vi "Read PWM Ratio.vi"(8 "error in (no error)":errorcluster, 11 "Set Ratio Msg in":refnum<class "Set Ratio Msg.lvclass">) -> (0 "error out":errorcluster, 2 "PWM Ratio":dbl format="%.3g", 3 "Set Ratio Msg out":refnum<class "Set Ratio Msg.lvclass">)   [LabVIEW 2017, in "BNT_DAQmx.lvlib" / "Set Ratio Msg.lvclass"]
uses:
  Set Ratio Msg.lvclass
  Set Ratio Msg.lvclass/Set Ratio Msg.ctl
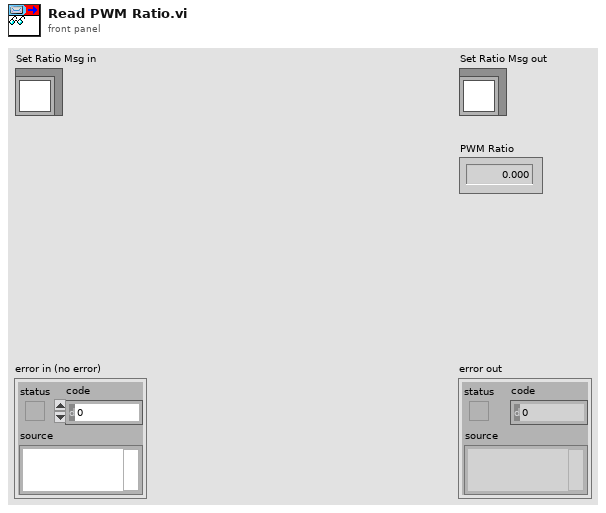
[diagram p1: front panel]
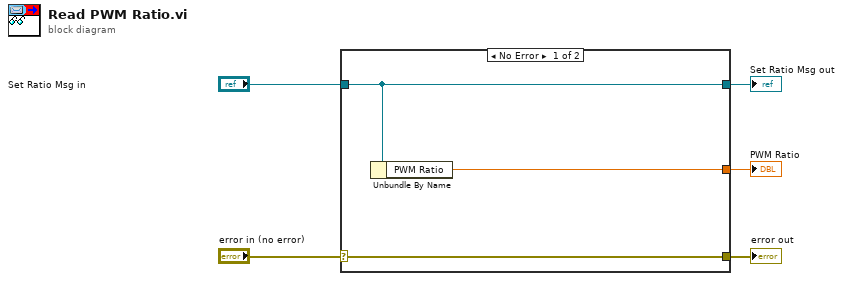
[diagram p0: block diagram]
diagram:
  n1 = case shown="No Error" "error in (no error)" {
    selector: "error in (no error)" -> [w8 w9]
    tunnel: [w8 w9] -> w4
    tunnel: [w7 w10] -> w2
    tunnel: "Set Ratio Msg in" -> [w7 w10]
    tunnel: [w6 _] -> w1
    frame No Error {
      n2 = Unbundle By Name(w7) -> ("PWM Ratio"=w6:dbl)
    }
    frame Error {
    }
  }
  "error out" <- w4
  "Set Ratio Msg out" <- w2
  "PWM Ratio" <- w1
